vi "Get Child Nodes.vi"(8 "error in":errorcluster, 11 "XML Document in":refnum<class "XML Document.lvclass">) -> (0 "error out":errorcluster, 3 "XML Document out":refnum<class "XML Document.lvclass">)   [LabVIEW 2014, in "XML Document.lvclass"]
uses:
  XML Document.lvclass
  Element_class/Element.lvclass
panel:
  out "Child Elements":refnum<class "Element.lvclass">[](array[class])
  in  "Element.lvclass":refnum<class "Element.lvclass">
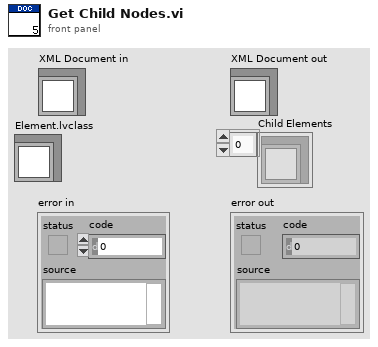
[diagram p1: front panel]
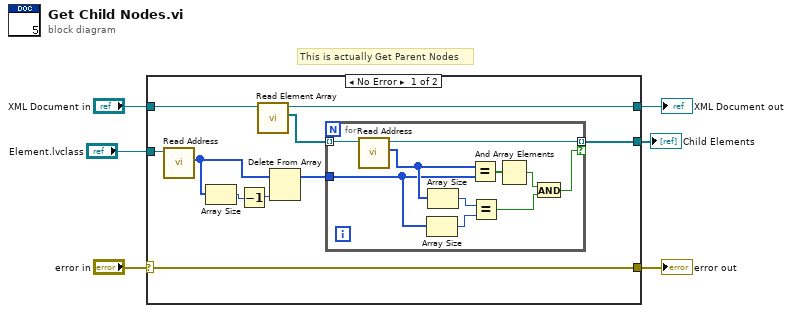
[diagram p0: block diagram]
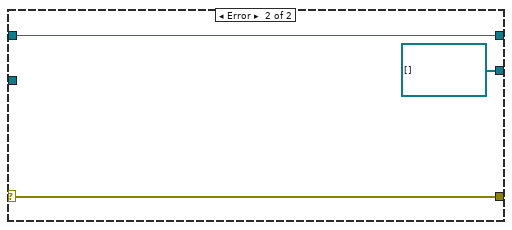
[diagram p2: hidden frame]
diagram:
  # "This is actually Get Parent Nodes"
  n1 = case shown="No Error" "error in" {
    selector: "error in" -> [w15 w29]
    tunnel: [w15 w29] -> w5
    tunnel: [w13 w28] -> w3
    tunnel: "XML Document in" -> [w16 w28]
    tunnel: "Element.lvclass" -> [w14 _]
    tunnel: [w7 refnum<class "Element.lvclass">[] []] -> w1
    frame No Error {
      n2 = call-dynamic "Read Address.vi"("Node in"=w14) -> ("Address"=w11:i32[])  [unwired: 8 in, 2 out]
      n3 = Array Size(array=w11) -> (size(s)=w9:i32)
      n4 = Decrement(x=w9) -> (x-1=w10:i32)
      n5 = call-dynamic "Read Element Array.vi"("XML Document in"=w16) -> ("Element Array"=w12:refnum<class "Element.lvclass">[], "XML Document out"=w13:refnum<class "XML Document.lvclass">)  [unwired: 8 in, 1 out]
      n6 = Delete From Array(array=w11, index=w10) -> (array with subset deleted=w8:i32[])  [unwired: 1 in, 1 out]
      n7 = for {
        tunnel: w12 -> [w26] mode=indexing
        tunnel: [w25] -> w7 mode=indexing if=w17
        tunnel: w8 -> [w23]
        n8 = call-dynamic "Read Address.vi"("Node in"=w26) -> ("Address"=w24:i32[], "Node out"=w25:refnum<class "Element.lvclass">)  [unwired: 8 in, 1 out]
        n9 = Array Size(array=w23) -> (size(s)=w20:i32)
        n10 = Array Size(array=w24) -> (size(s)=w21:i32)
        n11 = Equal?(x=w24, y=w23) -> (x = y?=w22:bool[])
        n12 = Equal?(x=w21, y=w20) -> (x = y?=w19:bool)
        n13 = And Array Elements(Boolean array=w22) -> (logical AND=w18:bool)
        n14 = And(x=w18, y=w19) -> (x .and. y?=w17:bool)
      }
    }
    frame Error {
    }
  }
  "error out" <- w5
  "XML Document out" <- w3
  "Child Elements" <- w1
